vi "niUSRP EX FSK Tx - 副本.vi"() -> ()   [LabVIEW 2015]
doc: "This example <B>requires the Modulation Toolkit</B>.\n\nApplies Frequency Shift Keying (FSK) to a PN sequence for USRP-based transmission. Continuously transmits a repeating message with a length determined by the PN Sequence Order parameter. \n\nThe example can generate FSK formats including 2-, 4-, 8-, and 16-FSK. It applies a pulse-shaping filter to the message signal, resamples the data to suit the timing specifications of the AWG, and ensures phase continuity in the data. \n\nYou can adjust the Digital Up Converter (DUC) Pre-Filter Gain to avoid overflow."
uses:
  <vilib>/measure/maspectr.llb/Power Spectrum and PSD Export Mode.ctl
  <vilib>/addons/Modulation/Digital/General/MT Generate FSK System Parameters(M).vi
  <instrlib>/niUSRP/niUSRP Write Tx Data (CDB Cluster).vi
  <vilib>/addons/Modulation/niDMT.lvlib
  <vilib>/measure/NI_MAPro.lvlib
panel:
  out "星座图":cluster{"x":dbl[], "x 2":dbl[]}(graph)
  in  "export mode":T1 caption="导出模式" items=["功率谱", "功率谱密度"]
  in  "Pulse Shaping Filter Parameters":T2={"Alpha"=0.5, "Filter Length"=6, "TX Filter"=enum."Root Raised Cos"} caption="Pulse Shaping Filter" {"Alpha" format="%.2f"}
  out "power spectrum":cluster{"f0":dbl, "df":dbl, "magnitude":dbl[]}(graph)={"f0"=-99999.99999999999, "df"=9.784735812133071, "magnitude"=array[20440 elements]} caption="Power Spectrum"
  in  "Enabled Channel":string(combo)="0"
  out "Tx Gain [dB] (actual)":dbl format="%#.6p"
  out "Tx Frequency \n[Hz] (actual)":dbl=467449999.9887113 format="%#.6p"
  out "Tx IQ Sampling\nRate [S/sec] (actual)":dbl=200000.0 format="%#.6p"
  in  "Active Antenna":string(combo)="TX1"
  in  "Tx Gain [dB]":dbl format="%#.6p"
  in  "Tx Frequency\n[Hz]":dbl=467450000.0 format="%#.6p"
  in  "Tx IQ Sampling\nRate [S/sec]":dbl=200000.0 format="%#.6p"
  in  "Device Name":refnum<k15>="192.168.10.2"
  in  "Fsk M-Ary":T3(ring)
  out "Signal Bandwidth [Hz]":dbl=25000.0 format="%#.2p"
  in  "Specify Mode":T4(tab)=enum."Specify FSK Deviation"
  in  "Modulation Index":dbl=0.3 format="%.2f"
  in  "FSK Deviation":dbl=50000.0 format="%#.4p"
  out "Generating?":bool
  in  "Stop":bool
  in  "Samples Per Symbol":i32=20
  out "Symbol Rate [Hz]":dbl=10000.0 format="%#.2p"
  in  "Pn Sequence Order":i32=9 min=5 max=16 step=1
  out "error out":errorcluster
  out "Frequency Deviation [Hz]":dbl=5000.0 format="%#.4p"
  # "FSK  Parameters"
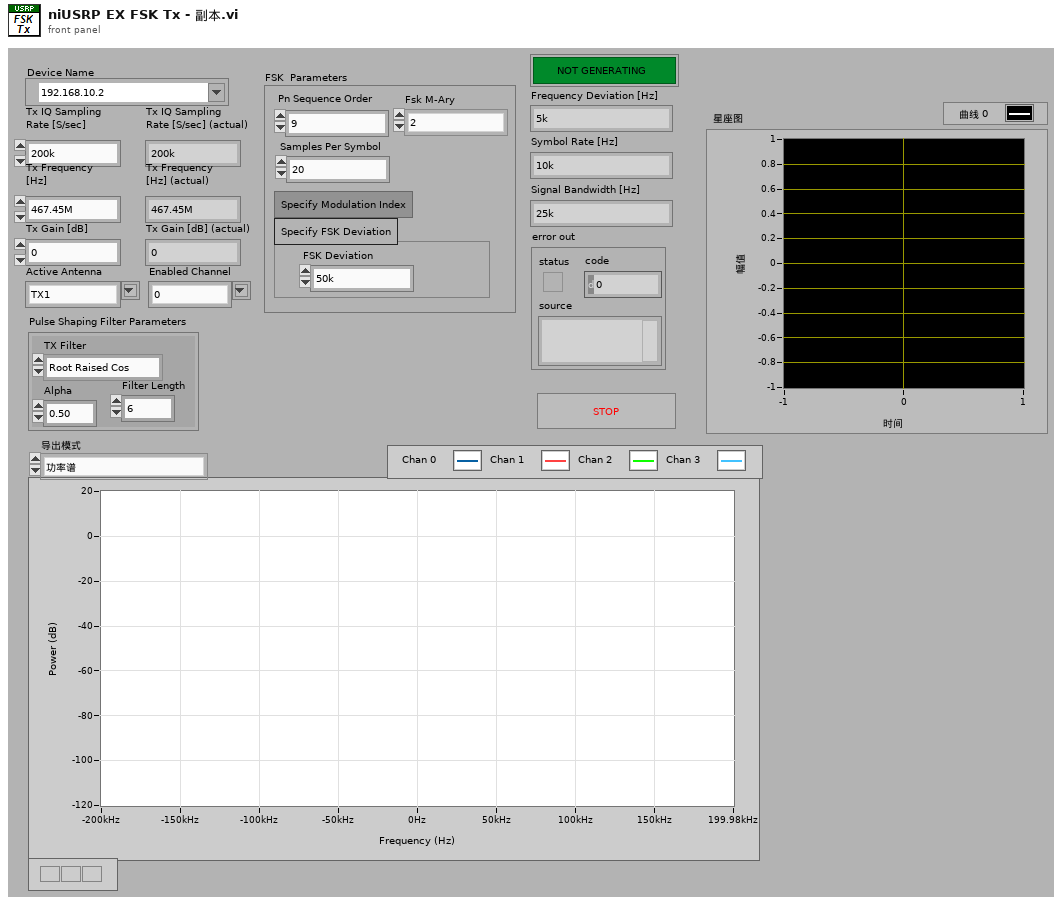
[diagram p1: front panel]
types:
  T1 = typedef "NI_MAPro.lvlib/Power Spectrum and PSD Export Mode.ctl" = u16
  T2 = cluster{"Alpha":dbl, "Filter Length":i32, "TX Filter":enum16{"none", "Raised Cosine", "Root Raised Cos", "Gaussian"}}
  T3 = enum16{"2", "4", "8", "16", "32", "64", "128", "256"}
  T4 = enum32{"Specify Modulation Index", "Specify FSK Deviation"}
  T5 = enum16{"none", "Raised Cosine", "Root Raised Cos", "Gaussian"}
  T6 = cluster{"samples per symbol (16)":i32, "symbol map":dbl[], "symbol phase continuity":enum16{"continuous", "discontinuous"}}
  T7 = typedef "niAMT.lvlib/Complex Data Waveform.ctl" = cluster{"t0":dbl, "dt":dbl, "Y":cdb[]}
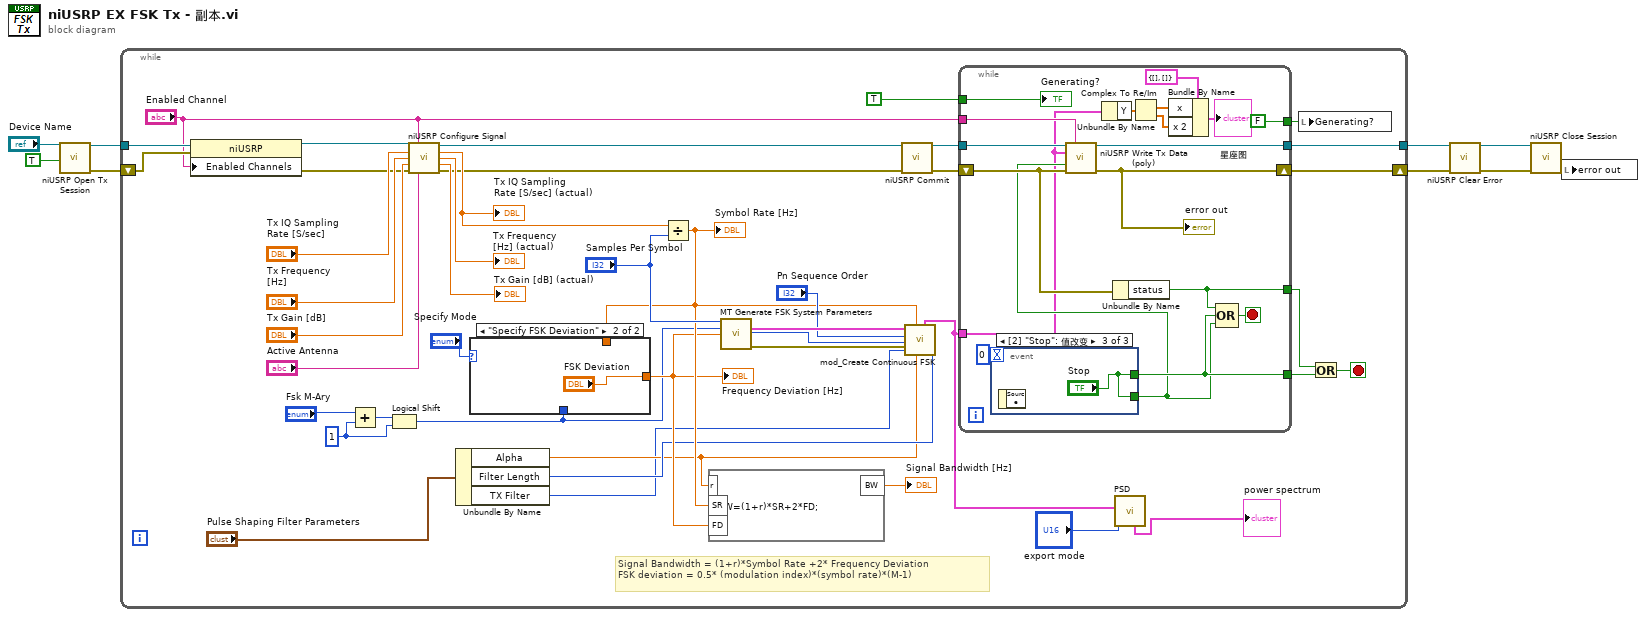
[diagram p0: block diagram]
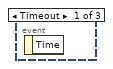
[diagram p2: hidden frame]
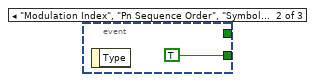
[diagram p3: hidden frame]
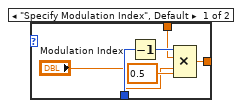
[diagram p4: hidden frame]
diagram:
  n1 = call <instrlib>:"niUSRP Open Tx Session.vi"("device names"="Device Name", "reset"=TRUE) -> ("session handle out"=w6:refnum<k15>, "error out"=w5:errorcluster)  [unwired: 12 in]
  n2 = while {
    tunnel: w6 -> [w18]
    tunnel: [w31] -> w4
    shift-right: [w45] -> w3
    shift-left: w5 -> [w17]
    stop <- w50 stop-if-true
    w41 = 1
    # "Signal Bandwidth = (1+r)*Symbol Rate +2* Frequency Deviation\nFSK deviation = 0.5* (modulation index)*(symbol rate)*(M-1)"
    n3 = property class="niUSRP"(reference=w18, error in=w17, "Enabled Channels"="Enabled Channel") -> (reference out=w16:refnum<k15>, error out=w15:errorcluster)
    n4 = Add(x="Fsk M-Ary", y=w41) -> (x+y=w42:i32)
    n5 = Logical Shift(y=w42, x=w41) -> (x << y=w24:i32)
    n6 = call <instrlib>:"niUSRP Configure Signal.vi"("session handle"=w16, "channel list"="Enabled Channel", "IQ rate"="Tx IQ Sampling\nRate [S/sec]", "carrier frequency"="Tx Frequency\n[Hz]", "gain"="Tx Gain [dB]", "error in (no error)"=w15, "active antenna"="Active Antenna") -> ("session handle out"=w22:refnum<k15>, "coerced IQ rate"=w23:dbl, "coerced carrier frequency"=→"Tx Frequency \n[Hz] (actual)":dbl, "coerced gain"=→"Tx Gain [dB] (actual)":dbl, "error out"=w21:errorcluster)  [unwired: 4 in]
    "Tx IQ Sampling\nRate [S/sec] (actual)" <- w23
    n7 = Unbundle By Name("Pulse Shaping Filter Parameters") -> ("Alpha"=w34:dbl, "Filter Length"=w35:i32, "TX Filter"=w33:T5)
    n8 = Divide(x=w23, y="Samples Per Symbol") -> (x/y=w39:dbl)
    "Symbol Rate [Hz]" <- w39
    n9 = case shown="\"Specify FSK Deviation\"" "Specify Mode" {
      tunnel: w39 -> [w77 _]
      tunnel: [w76 "FSK Deviation"] -> w38
      tunnel: w24 -> [w74 _]
      frame "Specify Modulation Index", Default {
        n10 = Decrement(x=w74) -> (x-1=w78:i32)
        n11 = Compound Arithmetic op=MULTIPLY(w78, w77, "Modulation Index", 0.5 ("value")) -> (w76:dbl)
      }
      frame "Specify FSK Deviation" {
      }
    }
    "Frequency Deviation [Hz]" <- w38
    n12 = formula code="BW=(1+r)*SR+2*FD;"("r"=w34, "SR"=w39, "FD"=w38) -> ("BW"=→"Signal Bandwidth [Hz]":dbl)
    n13 = call-poly <vilib>:"MT Generate FSK System Parameters.vi"("samples per symbol (16)"="Samples Per Symbol", "M-FSK (2)"=w24, "FSK deviation (Hz)"=w38) -> ("FSK system parameters"=w52:T6, "bits per symbol"=w49:i32, "error out"=w46:errorcluster)  [unwired: 10 in]
    n14 = call <instrlib>:"niUSRP Commit.vi"("session handle"=w22, "error in (no error)"=w21) -> ("session handle out"=w20:refnum<k15>, "error out"=w19:errorcluster)  [unwired: 12 in]
    n15 = call <vilib>:"mod_Create Continuous FSK.vi"("Filter Length"=w35, "TX Filter"=w33, "BT"=w34, "error in (no error)"=w46, "bits per symbol"=w49, "Symbol Rate, Hz"=w39, "PN Sequence Order"="Pn Sequence Order", "FSK system parameters"=w52) -> ("output complex waveform"=w12:T7)  [unwired: 2 out]
    n16 = while {
      shift-right: [w64] -> w45
      shift-left: w19 -> [w61]
      tunnel: [w62] -> w44
      tunnel: [w68] -> w51
      tunnel: w12 -> [w53]
      tunnel: TRUE ("Generating?") -> [w67]
      tunnel: [FALSE ("Generating?")] -> w36
      tunnel: w20 -> [w65]
      tunnel: [w63] -> w31
      tunnel: "Enabled Channel" -> [w59]
      stop <- w70 stop-if-true
      n17 = event shown="[2] \"Stop\": 值改变" {
        selector: _ -> [_ _ _]
        dyn-events: _ -> [_ _ _]
        timeout: 0 -> [_ _ _]
        tunnel: [_ TRUE "Stop"] -> w60
        tunnel: [_ _ "Stop"] -> w62
        event Timeout {
          n18 = event-data() -> ()  [unwired: 1 in, 1 out]
        }
        event "Modulation Index", "Pn Sequence Order", "Symbol Rate [Hz]", "Samples Per Symbol", "Specify Mode", "Fsk M-Ary", "Tx Frequency\n[Hz]", "Tx IQ Sampling\nRate [S/sec]", "Tx Gain [dB]", "Active Antenna", "FSK Deviation": Value Change {
          n19 = event-data() -> ()  [unwired: 1 in, 1 out]
        }
        event "Stop": Value Change {
          n20 = event-data() -> ()  [unwired: 1 in, 1 out]
        }
      }
      n21 = call-poly <instrlib>:"niUSRP Write Tx Data (poly).vi"("session handle"=w65, "channel list"=w59, "data"=w53, "end of data?"=w60, "error in (no error)"=w61) -> ("session handle out"=w63:refnum<k15>, "error out"=w64:errorcluster)  [unwired: 9 in]
      "error out" <- w64
      n22 = Unbundle By Name(w53) -> ("Y"=w58:cdb[])
      n23 = Unbundle By Name(w61) -> ("status"=w68:bool)
      n24 = Complex To Re/Im(x + iy=w58) -> (x=w55:dbl[], y=w56:dbl[])
      n25 = Bundle By Name(cluster=cluster{"x":dbl[], "x 2":dbl[]} {"x"=[], "x 2"=[]}, "x"=w55, "x 2"=w56) -> (→"星座图":cluster{"x":dbl[], "x 2":dbl[]})
      n26 = Compound Arithmetic op=OR(w68, w62, w60) -> (w70:bool)
      "Generating?" <- w67
    }
    n27 = call "PSD.vi"("output complex waveform"=w12, "export mode"="export mode") -> ("power spectrum"=→"power spectrum":cluster{"f0":dbl, "df":dbl, "magnitude":dbl[]})  [unwired: 8 in, 1 out]
    n28 = local write "Generating?"(w36) -> ()
    n29 = Or(x=w51, y=w44) -> (x .or. y?=w50:bool)
  }
  n30 = call <instrlib>:"niUSRP Clear Error.vi"("session handle"=w4, "error in (no error)"=w3) -> ("session handle out"=w2:refnum<k15>, "error out"=w1:errorcluster)  [unwired: 12 in]
  n31 = call <instrlib>:"niUSRP Close Session.vi"("session handle"=w2, "error in (no error)"=w1) -> ("error out"=w9:errorcluster)  [unwired: 13 in]
  n32 = local write "error out"(w9) -> ()
